vi "Filter DeBounce.vi"(6 "Reset":bool, 7 "Enable":bool=TRUE, 8 "error in (no error)":errorcluster caption="错误输入（无错误）", 10 "Filter Length":i32=10, 11 "Input":bool) -> (0 "error out":errorcluster caption="错误输出", 3 "Output":bool)   [LabVIEW 2012]
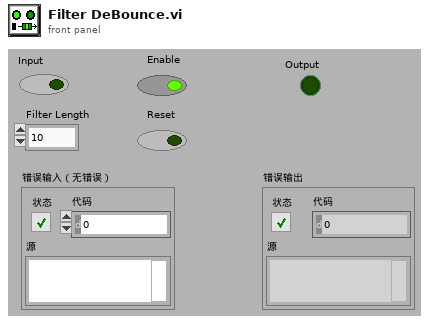
[diagram p1: front panel]
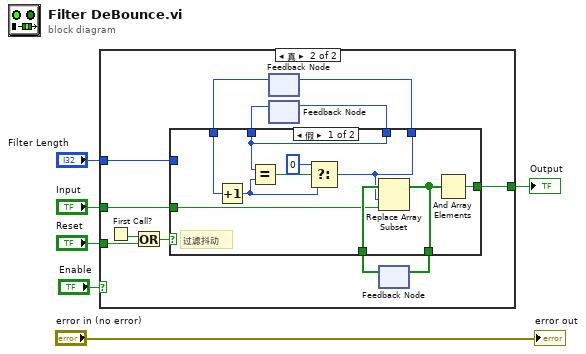
[diagram p0: block diagram]
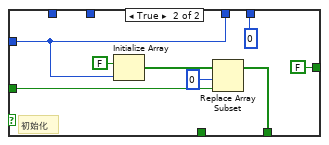
[diagram p3: hidden frame]
diagram:
  n1 = case shown="真" "Enable" {
    tunnel: [w7 w19] -> w6
    tunnel: "Input" -> [w7 w18]
    tunnel: "Filter Length" -> [_ w17]
    tunnel: "Reset" -> [_ w10]
    frame False {
    }
    frame True {
      n2 = First Call?() -> (First Call?: T/F=w9:bool)
      n3 = Or(x=w9, y=w10) -> (x .or. y?=w8:bool)
      n4 = feedback #1() -> (w13:i32)  [unwired: 1 in]
      n5 = feedback #2() -> (w12:i32)  [unwired: 1 in]
      n6 = feedback #3() -> (w11:bool[])  [unwired: 1 in]
      n7 = case shown="假" w8 {
        tunnel: w17 -> [_ w35]
        tunnel: [w22 w33] -> w16
        tunnel: [w20 w35] -> w15
        tunnel: [w24 0] -> w14
        tunnel: w13 -> [w29 _]
        tunnel: w12 -> [w20 _]
        tunnel: w11 -> [w25 _]
        tunnel: w18 -> [w23 w32]
        tunnel: [w21 FALSE] -> w19
        frame False {
          # "过滤抖动"
          n8 = Increment(x=w29) -> (x+1=w27:i32)
          n9 = Equal?(x=w20, y=w27) -> (x = y?=w28:bool)
          n10 = Select(t=0, s=w28, f=w27) -> (s? t:f=w24:i32)
          n11 = Replace Array Subset(array=w25, new element=w23, index=w24) -> (w22:bool[])
          n12 = And Array Elements(Boolean array=w22) -> (logical AND=w21:bool)
        }
        frame True {
          # "初始化"
          n13 = Initialize Array(FALSE, w35) -> (w37:bool[])
          n14 = Replace Array Subset(array=w37, new element=w32, index=0) -> (w33:bool[])
        }
      }
      n15 = feedback-in #1(w14) -> ()
      n16 = feedback-in #2(w15) -> ()
      n17 = feedback-in #3(w16) -> ()
    }
  }
  "Output" <- w6
  "error out" <- "error in (no error)"
